vi "Acquisition Message Loop.vi"(8 "error in (no error)":cluster{"状态":bool, "代码":i32, "源":string} caption="错误输入（无错误）", 9 "数据队列":refnum<queue>, 10 "数据通知器":refnum<notifier>, 11 "消息队列":T1) -> (0 "error out":cluster{"状态":bool, "代码":i32, "源":string} caption="错误输出")   [LabVIEW 2012, in "Acquisition.lvlib"]
doc: "该消息循环负责处理硬件数据采集的相关消息。"
uses:
  Acquisition.lvlib
  support/Message Queue/All Message Queues.ctl
  support/Message Queue/Message Cluster.ctl
  Hardware Configuration.ctl
  Signal Type.ctl
  support/Message Queue/Message Queue.lvlib
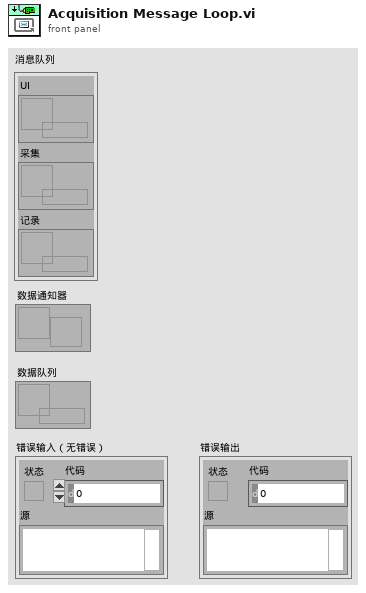
[diagram p1: front panel]
types:
  T1 = typedef "Message Queue.lvlib/All Message Queues.ctl" = cluster{"UI":refnum<queue>, "采集":refnum<queue>, "记录":refnum<queue>}
  T2 = typedef "Acquisition.lvlib/Hardware Configuration.ctl" = cluster{"硬件引用句柄<替换此项>":string, "信号类型<替换该项>":T3, "VISA资源名称":refnum<visa-resource-name>}
  T3 = typedef "Acquisition.lvlib/Signal Type.ctl" = enum16{"Sine Wave", "Square with Noise"}
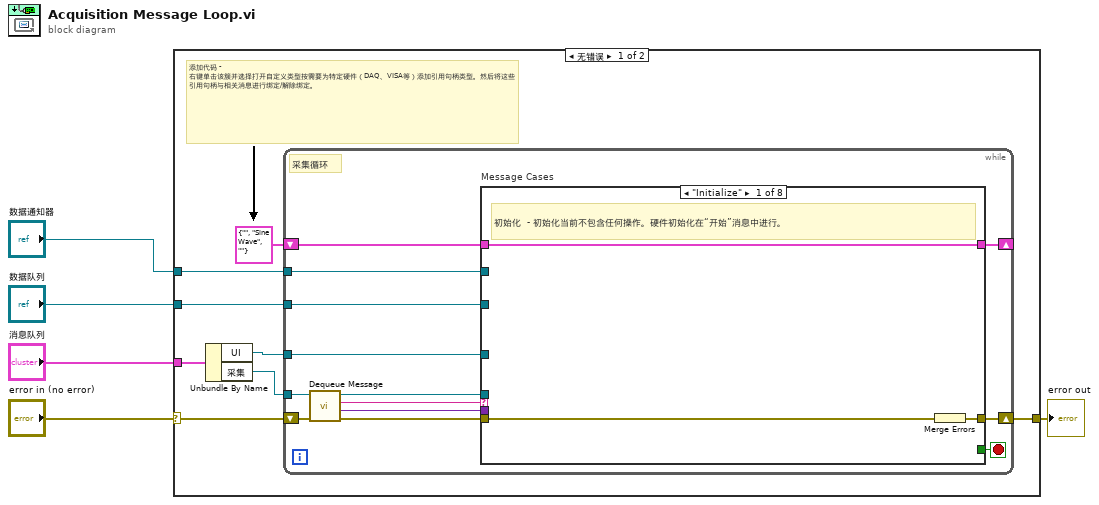
[diagram p0: block diagram]
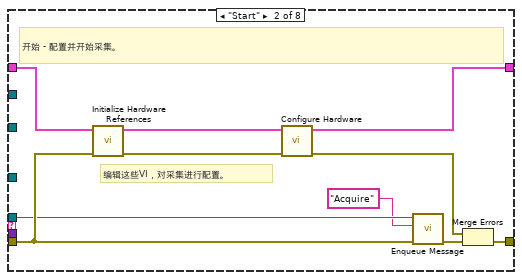
[diagram p2: hidden frame]
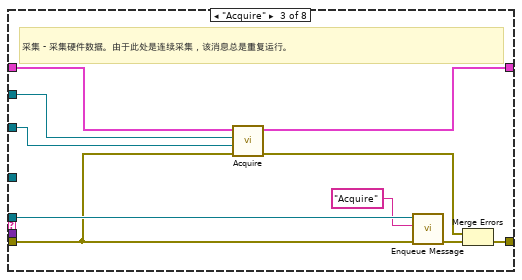
[diagram p3: hidden frame]
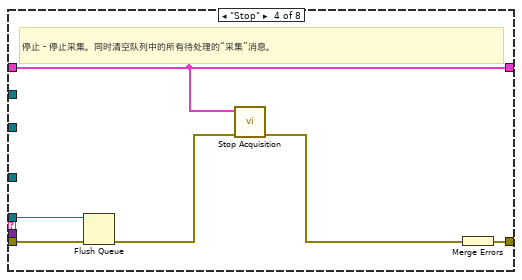
[diagram p4: hidden frame]
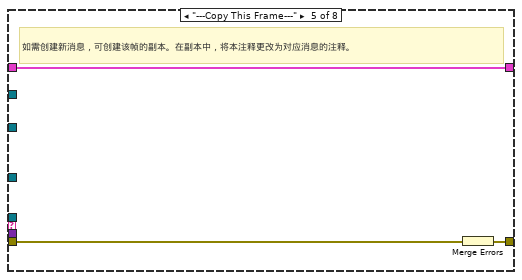
[diagram p5: hidden frame]
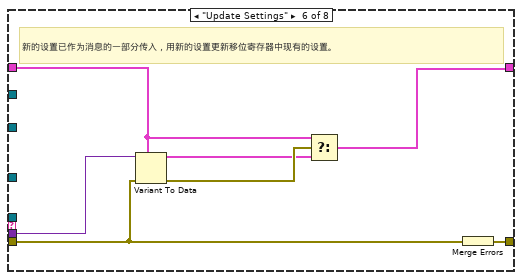
[diagram p6: hidden frame]
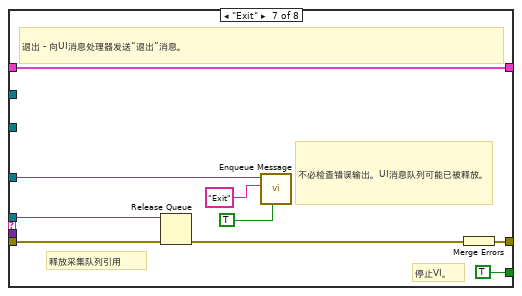
[diagram p7: hidden frame]
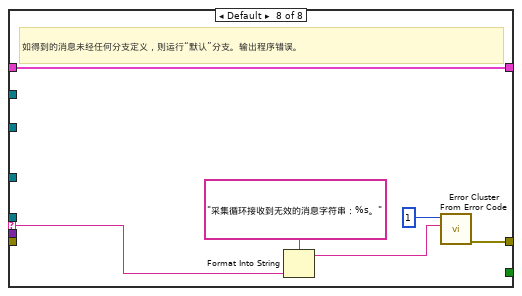
[diagram p8: hidden frame]
diagram:
  n1 = case shown="无错误" "error in (no error)" {
    selector: "error in (no error)" -> [w9 w81]
    tunnel: "消息队列" -> [w13 _]
    tunnel: [w11 w81] -> w4
    tunnel: "数据通知器" -> [w7 _]
    tunnel: "数据队列" -> [w6 _]
    frame No Error {
      # "添加代码 - 右键单击该簇并选择打开自定义类型按需要为特定硬件（DAQ、VISA等）添加引用句柄类型。然后将这些引用句柄与相关消息进行绑定/解除绑定。"
      n2 = Unbundle By Name(w13) -> ("UI"=w8:refnum<queue>, "采集"=w12:refnum<queue>)
      n3 = while {
        tunnel: w12 -> [w17]
        shift-right: [w25] -> _
        shift-left: T2 {"硬件引用句柄<替换此项>"="", "信号类型<替换该项>"=enum."Sine Wave", "VISA资源名称"=""} ("Data Cluster") -> [w26]
        shift-right: [w23] -> w11
        shift-left: w9 -> [w22]
        tunnel: w8 -> [w16]
        tunnel: w7 -> [w15]
        tunnel: w6 -> [w14]
        stop <- w24 stop-if-true
        # "采集循环"
        n4 = call "Dequeue Message.vi"("error in (no error)"=w22, "消息队列"=w17) -> ("error out"=w21:cluster{"状态":bool, "代码":i32, "源":string}, "消息数据"=w19:variant, "消息"=w20:string, "消息队列副本"=w18:refnum<queue>)  [unwired: 6 in]
        n5 = case "Message Cases" shown="\"Initialize\"" w20 {
          selector: w20 -> [_ _ _ _ _ _ _ w78]
          tunnel: w18 -> [_ w35 w47 w50 _ _ w66 _]
          tunnel: w21 -> [w28 w37 w46 w54 w58 w59 w70 _]
          tunnel: [w29 w39 w49 w55 w56 w65 w73 w76] -> w23
          tunnel: w26 -> [w27 w38 w43 w52 w57 w61 w72 w80]
          tunnel: [w27 w31 w44 w52 w57 w60 w72 w80] -> w25
          tunnel: [_ _ _ _ _ _ TRUE _] -> w24
          tunnel: w19 -> [_ _ _ _ _ w64 _ _]
          tunnel: w16 -> [_ _ _ _ _ _ w71 _]
          tunnel: w15 -> [_ _ w41 _ _ _ _ _]
          tunnel: w14 -> [_ _ w40 _ _ _ _ _]
          frame "Initialize" {
            # "初始化  - 初始化当前不包含任何操作。硬件初始化在“开始”消息中进行。"
            n6 = Merge Errors(w28) -> (w29:errorcluster)
          }
          frame "Start" {
            # "编辑这些VI，对采集进行配置。"
            # "开始 - 配置并开始采集。"
            n7 = call "Initialize Hardware References.vi"("error in (no error)"=w37, "硬件资源输入"=w38) -> ("error out"=w34:cluster{"状态":bool, "代码":i32, "源":string}, "硬件资源输出"=w32:T2)  [unwired: 8 in]
            n8 = call "Configure Hardware.vi"("error in (no error)"=w34, "硬件资源输入"=w32) -> ("error out"=w33:cluster{"状态":bool, "代码":i32, "源":string}, "硬件资源输出"=w31:T2)  [unwired: 8 in]
            n9 = call "Enqueue Message.vi"("error in (no error)"=w37, "消息"="Acquire" ("Message"), "消息队列"=w35) -> ("error out"=w36:cluster{"状态":bool, "代码":i32, "源":string})  [unwired: 7 in, 1 out]
            n10 = Merge Errors(w33, w36) -> (w39:errorcluster)
          }
          frame "Acquire" {
            # "采集 - 采集硬件数据。由于此处是连续采集，该消息总是重复运行。"
            n11 = call "Acquire.vi"("error in (no error)"=w46, "数据队列"=w40, "数据通知器"=w41, "硬件资源输入"=w43) -> ("error out"=w45:cluster{"状态":bool, "代码":i32, "源":string}, "硬件资源输出"=w44:T2)  [unwired: 6 in]
            n12 = call "Enqueue Message.vi"("error in (no error)"=w46, "消息"="Acquire" ("Message"), "消息队列"=w47) -> ("error out"=w48:cluster{"状态":bool, "代码":i32, "源":string})  [unwired: 7 in, 1 out]
            n13 = Merge Errors(w45, w48) -> (w49:errorcluster)
          }
          frame "Stop" {
            # "停止 - 停止采集。同时清空队列中的所有待处理的“采集”消息。"
            n14 = Flush Queue(queue=w50, error in (no error)=w54) -> (error out=w51:errorcluster)  [unwired: 2 out]
            n15 = call "Stop Acquisition.vi"("error in (no error)"=w51, "硬件资源输入"=w52) -> ("error out"=w53:cluster{"状态":bool, "代码":i32, "源":string})  [unwired: 9 in]
            n16 = Merge Errors(w53) -> (w55:errorcluster)
          }
          frame "---Copy This Frame---" {
            # "如需创建新消息，可创建该帧的副本。在副本中，将本注释更改为对应消息的注释。"
            n17 = Merge Errors(w58) -> (w56:errorcluster)
          }
          frame "Update Settings" {
            # "新的设置已作为消息的一部分传入，用新的设置更新移位寄存器中现有的设置。"
            n18 = Variant To Data(error in=w59, type=w61, Variant=w64) -> (data=w62:T2, error out=w63:errorcluster)
            n19 = Select(t=w61, s=w63, f=w62) -> (s? t:f=w60:T2)
            n20 = Merge Errors(w59) -> (w65:errorcluster)
          }
          frame "Exit" {
            # "不必检查错误输出。UI消息队列可能已被释放。"
            # "释放采集队列引用"
            # "停止VI。"
            # "退出 - 向UI消息处理器发送“退出”消息。"
            n21 = Release Queue(queue=w66, error in (no error)=w70) -> (error out=w67:errorcluster)  [unwired: 1 in, 2 out]
            n22 = call "Enqueue Message.vi"("优先消息？(F)"=TRUE, "消息"="Exit" ("Message"), "消息队列"=w71) -> ()  [unwired: 7 in, 2 out]
            n23 = Merge Errors(w67) -> (w73:errorcluster)
          }
          frame Default {
            # "如得到的消息未经任何分支定义，则运行“默认”分支。输出程序错误。"
            n24 = Format Into String(format string="采集循环接收到无效的消息字符串：%s。" ("Invalid Acquisition Message"), w78) -> (resulting string=w75:string)  [unwired: 2 in, 1 out]
            n25 = call <vilib>:"Error Cluster From Error Code.vi"("error message (\"\")"=w75, "error code (0)"=1) -> ("error out"=w76:errorcluster)  [unwired: 7 in]
          }
        }
      }
    }
    frame Error {
    }
  }
  "error out" <- w4
